vi "Score Ellipse.vi"(4 "Bottom":dbl, 5 "Area":dbl, 6 "Right":dbl, 7 "Height":dbl, 9 "Top":dbl, 10 "Left":dbl, 11 "Width":dbl) -> (1 "Y":dbl, 2 "X":dbl, 3 "Area %":dbl)   [LabVIEW 2012]
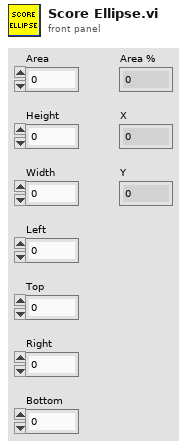
[diagram p1: front panel]
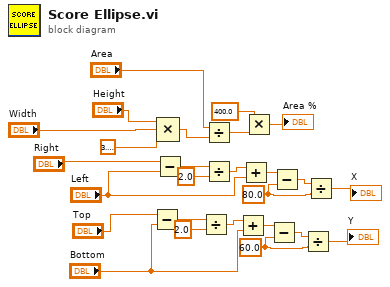
[diagram p0: block diagram]
diagram:
  w16 = 60.0 ("y")
  w15 = 80.0 ("y")
  n1 = Subtract(x="Top", y="Bottom") -> (x-y=w21:dbl)
  n2 = Subtract(x="Right", y="Left") -> (x-y=w8:dbl)
  n3 = Compound Arithmetic op=MULTIPLY("Height", "Width", 3.141592653589793) -> (w5:dbl)
  n4 = Divide(x=w21, y=2.0) -> (x/y=w19:dbl)
  n5 = Divide(x="Area", y=w5) -> (x/y=w6:dbl)
  n6 = Divide(x=w8, y=2.0) -> (x/y=w10:dbl)
  n7 = Add(x=w19, y="Bottom") -> (x+y=w18:dbl)
  n8 = Add(x=w10, y="Left") -> (x+y=w13:dbl)
  n9 = Multiply(x=400.0, y=w6) -> (x*y=→"Area %":dbl)
  n10 = Subtract(x=w18, y=w16) -> (x-y=w17:dbl)
  n11 = Subtract(x=w13, y=w15) -> (x-y=w14:dbl)
  n12 = Divide(x=w17, y=w16) -> (x/y=→"Y":dbl)
  n13 = Divide(x=w14, y=w15) -> (x/y=→"X":dbl)
